vi "DSF.Transceiver.UDP.Configuration.Initialize.vi"(8 "error in (no error)":errorcluster, 11 "UDP Configuration in":refnum<class "DSF.Transceiver.UDP.Configuration.lvclass">) -> (0 "error out":errorcluster, 3 "UDP Configuration out":refnum<class "DSF.Transceiver.UDP.Configuration.lvclass">)   [LabVIEW 2017, in "DSF.Transceiver.UDP.lvlib" / "DSF.Transceiver.UDP.Configuration.lvclass"]
uses:
  DSF.Transceiver.UDP.Configuration.lvclass
  DSF.Transceiver.UDP.Configuration.lvclass/DSF.Transceiver.UDP.Configuration.ctl
  Built/Windows/Engine/DSF.Engine.lvlibp/Shared/Classes/Configuration/DSF.Shared.Configuration.lvclass
  C:/Git/DSF/DSF Core/Built/Windows/Engine/DSF.Engine.lvlibp/Shared/Classes/Configuration/DSF.Shared.Configuration.lvclass
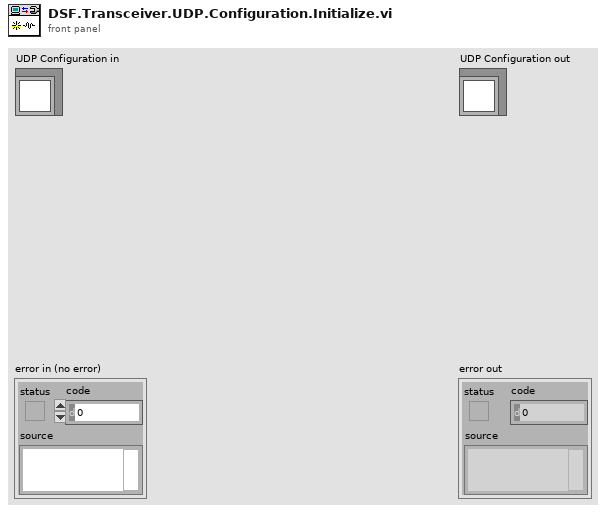
[diagram p1: front panel]
types:
  T1 = typedef "DSF.Engine.lvlibp/DSF Configuration API.lvlib/DSF Settings Info.ctl" = cluster{"key":string, "value":string}[]
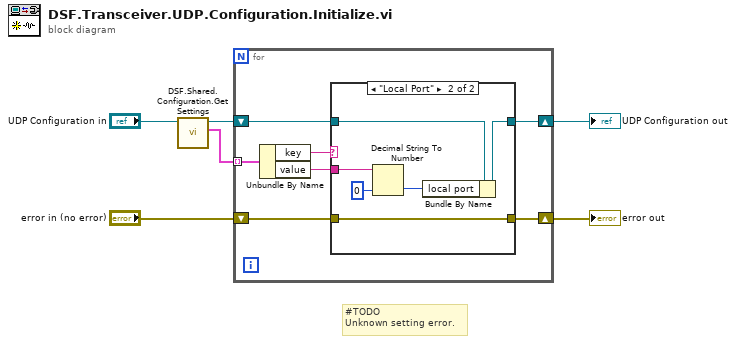
[diagram p0: block diagram]
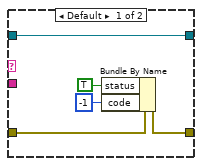
[diagram p2: hidden frame]
diagram:
  # "#TODO\nUnknown setting error."
  n1 = call "DSF.Shared.Configuration.Get Settings.vi"("Configuration in"="UDP Configuration in") -> ("settings"=w5:T1, "Configuration out"=w4:refnum<class "DSF.Transceiver.UDP.Configuration.lvclass">)  [unwired: 9 in]
  n2 = for {
    tunnel: w5 -> [w13] mode=indexing
    shift-right: [w9] -> w3
    shift-left: w4 -> [w10]
    shift-right: [w7] -> w1
    shift-left: "error in (no error)" -> [w8]
    n3 = Unbundle By Name(w13) -> ("key"=w12:string, "value"=w11:string)
    n4 = case shown="\"Local Port\"" w12 {
      tunnel: w11 -> [_ w23]
      tunnel: w10 -> [w18 w22]
      tunnel: [w18 w21] -> w9
      tunnel: w8 -> [w17 w19]
      tunnel: [w16 w19] -> w7
      frame Default {
        n5 = Bundle By Name(cluster=w17, "status"=TRUE, "code"=-1) -> (w16:errorcluster)
      }
      frame "Local Port" {
        n6 = Decimal String To Number(string=w23, default (0L)=u16 0 ("default (0 I32)")) -> (number=w20:u16)  [unwired: 1 in, 1 out]
        n7 = Bundle By Name(cluster=w22, "local port"=w20) -> (w21:refnum<class "DSF.Transceiver.UDP.Configuration.lvclass">)
      }
    }
  }
  "error out" <- w1
  "UDP Configuration out" <- w3
